vi "Script Wiki Page.vi"(8 "Error In":errorcluster, 10 "Relative Wiki Path":string="{{ ", 11 "VI Data":T1) -> (0 "Error Out":errorcluster, 3 "Wiki Page Syntax":string)   [LabVIEW 2014]
uses:
  VI Data.ctl
  Control Info.ctl
  <vilib>/picture/picture.llb/imagedata.ctl
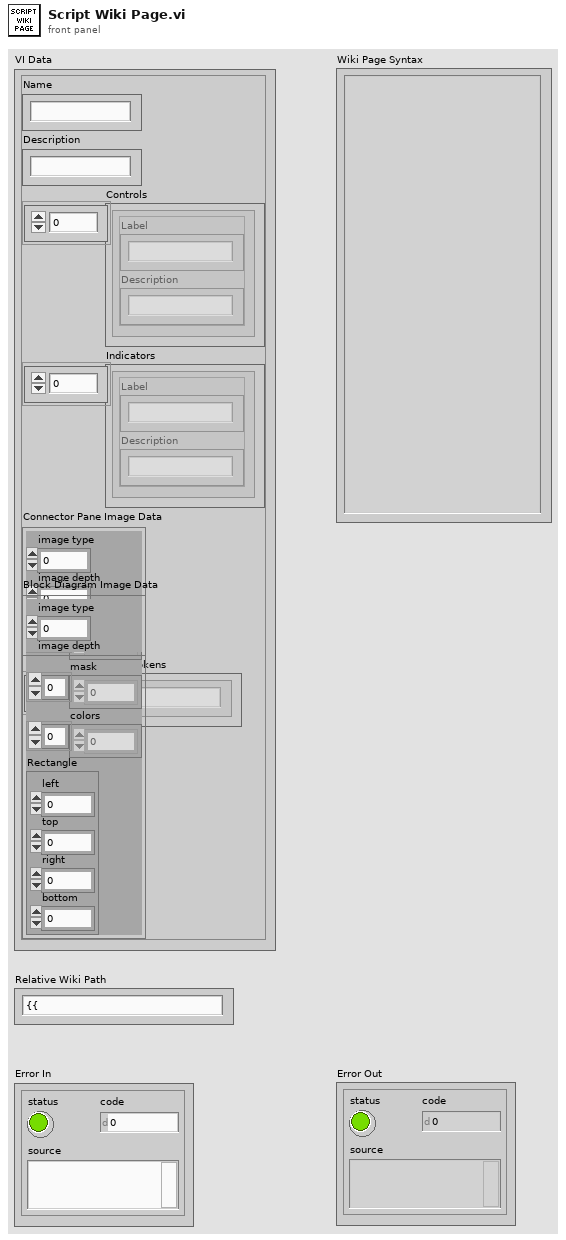
[diagram p1: front panel]
types:
  T1 = typedef "VI Data.ctl" = cluster{"Name":string, "Description":string, "Controls":T2[], "Indicators":T2[], "Connector Pane Image Data":T3, "Block Diagram Image Data":T3, "Path Tokens":string[]}
  T2 = typedef "Control Info.ctl" = cluster{"Label":string, "Description":string}
  T3 = typedef "imagedata.ctl" = cluster{"image type":i32, "image depth":i32, "image":u8[], "mask":u8[], "colors":u32[], "Rectangle":cluster{"left":i16, "top":i16, "right":i16, "bottom":i16}}
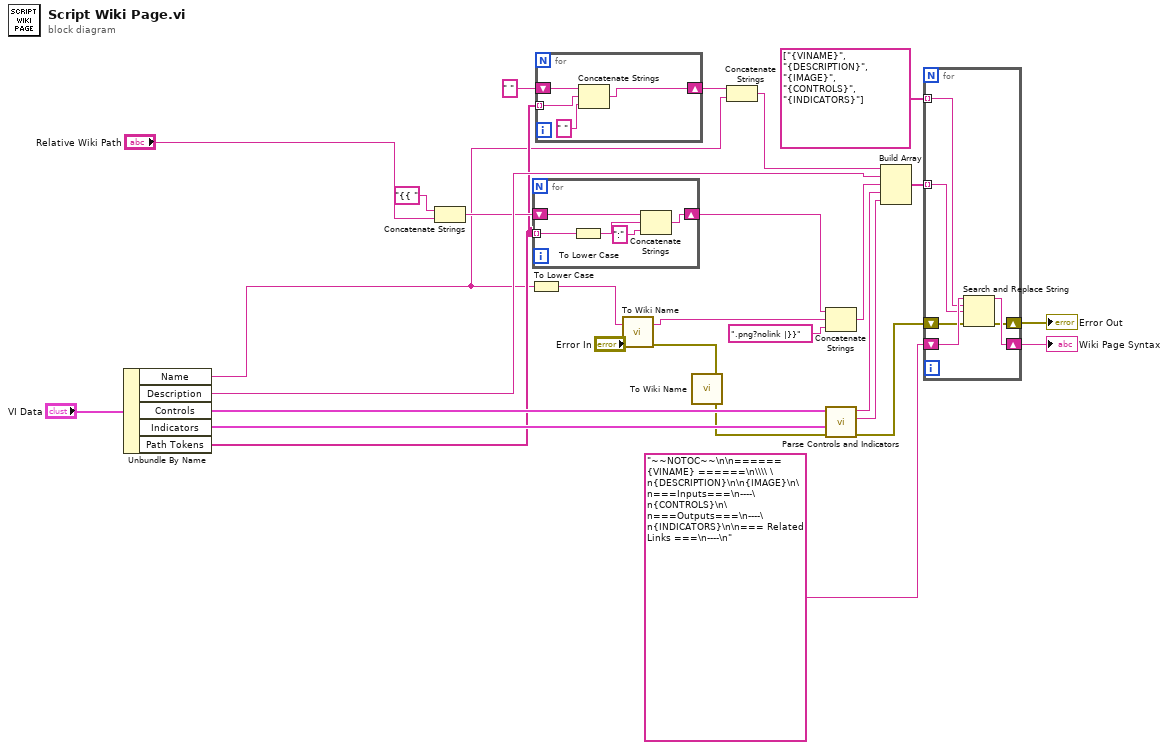
[diagram p0: block diagram]
diagram:
  n1 = Unbundle By Name("VI Data") -> ("Name"=w2:string, "Description"=w21:string, "Controls"=w17:T2[], "Indicators"=w12:T2[], "Path Tokens"=w5:string[])
  n2 = Concatenate Strings("{{ ", "Relative Wiki Path") -> (w9:string)
  n3 = To Lower Case(string=w2) -> (all lower case string=w6:string)
  n4 = for {
    tunnel: w5 -> [w28] mode=indexing
    shift-right: [w30] -> w14
    shift-left: w9 -> [w31]
    n5 = To Lower Case(string=w28) -> (all lower case string=w27:string)
    n6 = Concatenate Strings(w31, w27, ":" ("string")) -> (w30:string)
  }
  n7 = for {
    shift-right: [w33] -> w3
    shift-left: " " -> [w35]
    tunnel: w5 -> [w34] mode=indexing
    n8 = Concatenate Strings(w35, w34, " " ("string")) -> (w33:string)
  }
  n9 = call "To Wiki Name.vi"("Name"=w6) -> ("Wiki Name"=w7:string)  [unwired: 2 in]
  n10 = call "To Wiki Name.vi"() -> ()  [unwired: 3 in, 1 out]
  n11 = Concatenate Strings(w3, w2) -> (w1:string)
  n12 = Concatenate Strings(w14, w7, ".png?nolink |}}" ("string")) -> (w13:string)
  n13 = call "Parse Controls and Indicators.vi"("Error In"="Error In", "Indicators"=w12, "Controls"=w17) -> ("Error Out"=w19:errorcluster, "Indicators  Wiki Syntax"=w16:string, "Contorls Wiki Syntax"=w18:string)  [unwired: 6 in]
  n14 = Build Array(w1, w21, w13, w18, w16) -> (w20:string[])
  n15 = for {
    tunnel: string[] ["{VINAME}", "{DESCRIPTION}", "{IMAGE}", "{CONTROLS}", "{INDICATORS}"] -> [w40] mode=indexing
    tunnel: w20 -> [w39] mode=indexing
    shift-right: [w38] -> w24
    shift-left: "~~NOTOC~~\n\n====== {VINAME} ======\n\\\\ \n{DESCRIPTION}\n\n{IMAGE}\n\n===Inputs===\n----\n{CONTROLS}\n\n===Outputs===\n----\n{INDICATORS}\n\n=== Related Links ===\n----\n" ("format string") -> [w41]
    shift-right: [w37] -> w23
    shift-left: w19 -> [w36]
    n16 = Search and Replace String(input string=w41, search string=w40, replace string=w39, error in=w36) -> (result string=w38:string, error out=w37:errorcluster)  [unwired: 4 in, 2 out]
  }
  "Wiki Page Syntax" <- w24
  "Error Out" <- w23
